vi "ABB Set VT-CT Ratios.vi"(10 "Test name":string, 11 "VT and CT Ratios":T1) -> (3 "VT and CT Ratios out":T1)   [LabVIEW 2017]
panel:
  in  "exit":bool
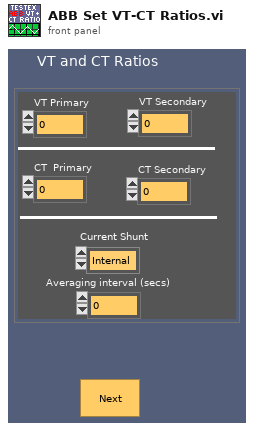
[diagram p1: front panel]
types:
  T1 = cluster{"VT Primary":dbl, "VT Secondary":dbl, "CT  Primary":dbl, "CT Secondary":dbl, "Current Shunt":enum16{"Internal", "External"}, "Averaging interval (secs)":dbl}
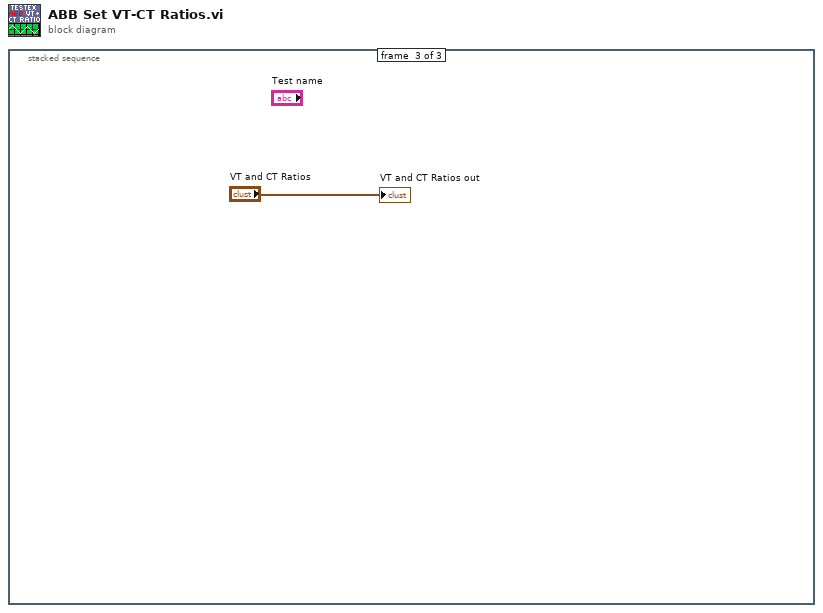
[diagram p0: block diagram]
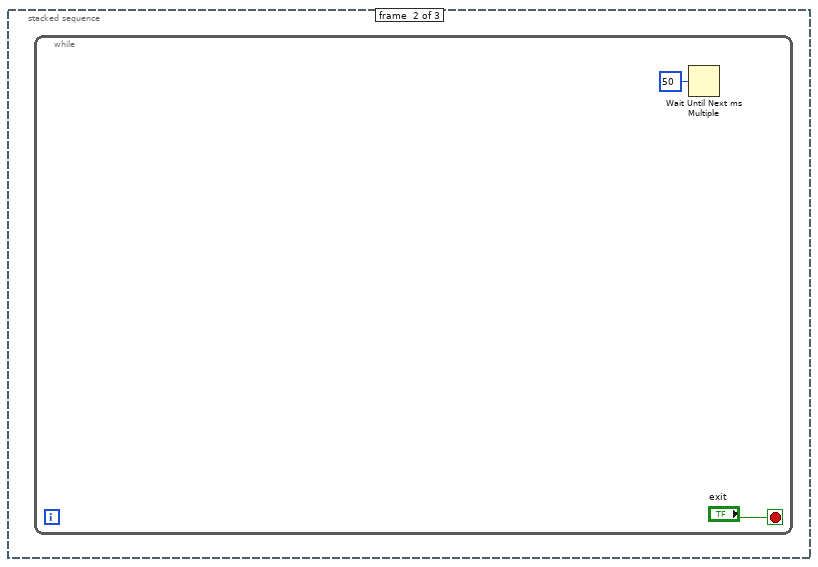
[diagram p3: hidden frame]
diagram:
  n1 = stacked-sequence {
    frame #0 {
    }
    frame #1 {
      n2 = while {
        stop <- "exit" stop-if-true
        n3 = Wait Until Next ms Multiple(millisecond multiple=u32 50) -> ()  [unwired: 1 out]
      }
    }
    frame #2 {
      "VT and CT Ratios out" <- "VT and CT Ratios"
    }
  }
